vi "BRig_Host__Loop_Consumer_RunState__updatePlot__v2.vi"(5 "input_idx":i32[](array[numeric]), 6 "input_DisplayNumber":u16, 7 "input_dataPlot":u16[][](array[numeric]), 11 "input_updatePlot":bool) -> (0 "output_X_min":dbl, 1 "output_X_max":dbl, 2 "output_X_inc":dbl, 3 "XY Graph":cluster{u16[], u16[]}[](graph))   [LabVIEW 2014]
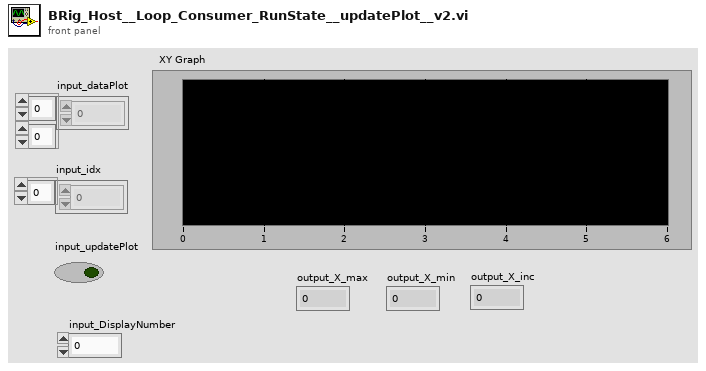
[diagram p1: front panel]
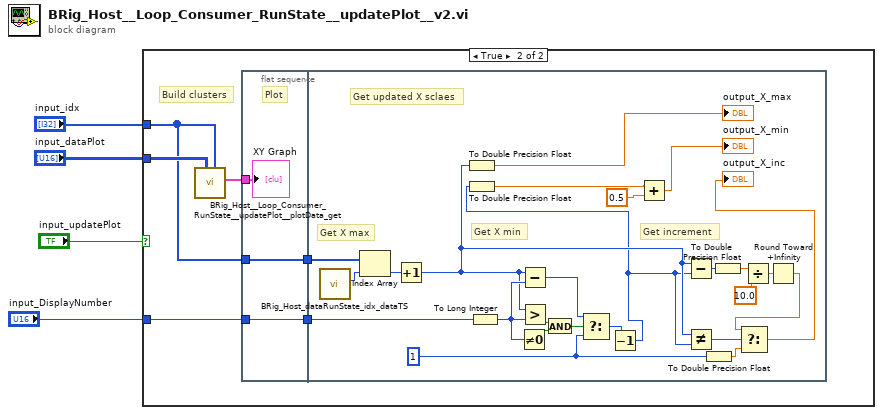
[diagram p0: block diagram]
diagram:
  n1 = case shown="True" "input_updatePlot" {
    tunnel: "input_idx" -> [_ w5]
    tunnel: "input_dataPlot" -> [_ w10]
    tunnel: "input_DisplayNumber" -> [_ w7]
    frame False {
    }
    frame True {
      # "Build clusters"
      n2 = call "BRig_Host__Loop_Consumer_RunState__updatePlot__plotData_get.vi"("input_idx"=w5, "input_dataPlot"=w10) -> ("output_plotData"=w9:cluster{u16[], u16[]}[])  [unwired: 9 in]
      n3 = flat-sequence {
        tunnel: w9 -> [w13]
        tunnel: [w12] -> w8
        tunnel: w7 -> [w12]
        tunnel: [w11] -> w6
        tunnel: w5 -> [w11]
        tunnel: w8 -> [w36]
        tunnel: w6 -> [w38]
        frame #0 {
          # "Plot"
          "XY Graph" <- w13
        }
        frame #1 {
          w24 = 1 ("t")
          # "Get increment"
          # "Get X min"
          # "Get X max"
          # "Get updated X sclaes"
          n4 = call "BRig_Host_dataRunState_idx_dataTS.vi"() -> ("output_idx_dataTS"=w37:i32)  [unwired: 11 in]
          n5 = Index Array(array=w38, index=w37) -> (element=w21:i32)
          n6 = Increment(x=w21) -> (x+1=w20:i32)
          n7 = To Double Precision Float(number=w20) -> (double precision float=→"output_X_max":dbl)
          n8 = To Long Integer(number=w36) -> (32bit integer=w33:i32)
          n9 = Not Equal To 0?(x=w33) -> (x != 0?=w35:bool)
          n10 = Subtract(x=w20, y=w33) -> (x-y=w29:i32)
          n11 = Greater?(x=w20, y=w33) -> (0:w34:bool)
          n12 = And(x=w34, y=w35) -> (x .and. y?=w32:bool)
          n13 = Select(t=w29, s=w32, f=w24) -> (s? t:f=w18:i32)
          n14 = Decrement(x=w18) -> (x-1=w17:i32)
          n15 = To Double Precision Float(number=w17) -> (double precision float=w15:dbl)
          n16 = Add(x=w15, y=0.5) -> (x+y=→"output_X_min":dbl)
          n17 = Subtract(x=w20, y=w17) -> (x-y=w31:i32)
          n18 = Not Equal?(x=w20, y=w17) -> (x != y?=w30:bool)
          n19 = To Double Precision Float(number=w24) -> (double precision float=w23:dbl)
          n20 = To Double Precision Float(number=w31) -> (double precision float=w27:dbl)
          n21 = Divide(x=w27, y=10.0) -> (x/y=w26:dbl)
          n22 = Round Toward +Infinity(x=w26) -> (ceil(x): smallest int >= x=w25:dbl)
          n23 = Select(t=w25, s=w30, f=w23) -> (s? t:f=→"output_X_inc":dbl)
        }
      }
    }
  }
